vi "NavX Gyro.vi"(10 "Reset":bool, 11 "Enum":T5) -> (2 "Status":T1 {"NAVX_OP_STATUS" items=["INITIALIZING", "SELFTEST_IN_PROGRESS", "ERROR", "IMU_AUTOCAL_IN_PROGRESS", "NORMAL"]; "NAVX_CAL_STATUS" items=["IMU_CAL_STATE_MASK"=3, "IMU_CAL_INPROGRESS"=0, "IMU_CAL_ACCUMULATE"=1, "IMU_CAL_COMPLETE"=2, "MAG_CAL_COMPLETE"=4, "BARO_CAL_COMPLETE"=8]}, 3 "Angle":dbl)   [LabVIEW 2014]
uses:
  TypeDefs/SRE Enum.ctl
  navX Gyroscope/COMMON/TypeDefs/Data TypeDefs/navX Status Data.ctl
  navX Gyroscope/COMMON/TypeDefs/Value TypeDefs/navX NAVX_OP_STATUS.ctl
  navX Gyroscope/COMMON/TypeDefs/Value TypeDefs/navX NAVX_CAL_STATUS.ctl
  navX Gyroscope/COMMON/TypeDefs/Value TypeDefs/navX NAVX_SENSOR_STATUS.ctl
  navX Gyroscope/COMMON/TypeDefs/Value TypeDefs/navX Update Rate.ctl
  navX Gyroscope/COMMON/TypeDefs/Value TypeDefs/navX Interface Protocol.ctl
  <vilib>/Rock Robotics/SystemInterfaces/i2clib/i2c_bus.ctl
  navX Gyroscope/navX-MXP IMU.lvlib
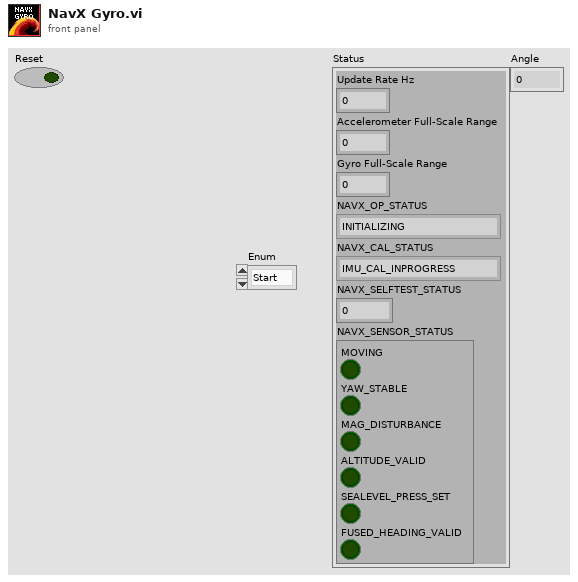
[diagram p1: front panel]
types:
  T1 = typedef "navX-MXP IMU.lvlib/navX Status Data.ctl" = cluster{"Update Rate Hz":u8, "Accelerometer Full-Scale Range":u8, "Gyro Full-Scale Range":u16, "NAVX_OP_STATUS":T2, "NAVX_CAL_STATUS":T3, "NAVX_SELFTEST_STATUS":u8, "NAVX_SENSOR_STATUS":T4}
  T2 = typedef "navX-MXP IMU.lvlib/navX NAVX_OP_STATUS.ctl" = u8
  T3 = typedef "navX-MXP IMU.lvlib/navX NAVX_CAL_STATUS.ctl" = u8
  T4 = typedef "navX-MXP IMU.lvlib/navX NAVX_SENSOR_STATUS.ctl" = cluster{"MOVING":bool, "YAW_STABLE":bool, "MAG_DISTURBANCE":bool, "ALTITUDE_VALID":bool, "SEALEVEL_PRESS_SET":bool, "FUSED_HEADING_VALID":bool}
  T5 = typedef "SRE Enum.ctl" = enum16{"Start", "Run", "End"}
  T6 = typedef "i2c_bus.ctl" = enum16{"I2C On-Board", "I2C MXP", "Invalid"}
  T7 = typedef "navX-MXP IMU.lvlib/navX Interface Protocol.ctl" = enum16{"SPI", "I2C"}
  T8 = typedef "navX-MXP IMU.lvlib/navX Update Rate.ctl" = u8
  T9 = typedef "navX-MXP IMU.lvlib/navX Device TypeDef.ctl" = cluster{"navX Interface Protocol":T7, "navX Interface Protocol TypeDefs":cluster{"SPIDevRef":T10, "I2CDevRef":T13}, "navX System Information":cluster{"Board Information":T14, "Status":T1, "Offsets":T15}, "navX Common Information":cluster{"Update Rate (4Hz-60Hz)":T8, "refnum name":string, "error":errorcluster}}
  T10 = typedef "WPI_SPIDevRef.ctl" = cluster{"DevStatus":errorcluster, "Handle":i32, "Controller":T11, "SPI Bus":T12}
  T11 = typedef "FPGA_TypedefDigitalModule.ctl" = enum16{"Controller 1"}
  T12 = typedef "spi_bus.ctl" = enum16{"SPI On-Board, CS0", "SPI On-Board, CS1", "SPI On-Board, CS2", "SPI On-Board, CS3", "SPI MXP", "Invalid"}
  T13 = typedef "WPI_I2CDevRef.ctl" = cluster{"DevStatus":errorcluster, "Controller":T11, "Device Address":u8, "Handle":i32, "I2C Bus":T6}
  T14 = typedef "navX-MXP IMU.lvlib/navX Board Information.ctl" = cluster{"WhoAmI (50 | 0x32)":u8, "Board Revision":u8, "Firmware Major Version":u8, "Firmware Minor Version":u8}
  T15 = typedef "navX-MXP IMU.lvlib/navX Offsets Data.ctl" = cluster{"Yaw":dbl, "Quat W":dbl, "Quat X":dbl, "Quat Y":dbl, "Quat Z":dbl}
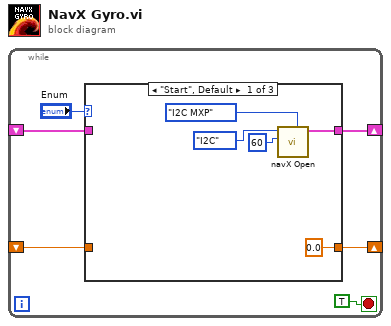
[diagram p0: block diagram]
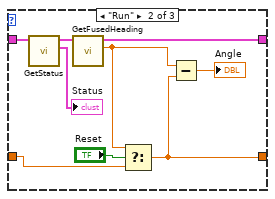
[diagram p2: hidden frame]
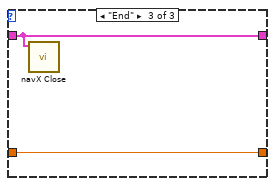
[diagram p3: hidden frame]
diagram:
  n1 = while {
    shift-right: [w4] -> _
    shift-left: _ -> [w3]
    shift-right: [w2] -> _
    shift-left: _ -> [w1]
    stop <- TRUE stop-if-true
    n2 = case shown="\"Start\", Default" "Enum" {
      tunnel: [w8 w18 w22] -> w4
      tunnel: w3 -> [_ w20 w22]
      tunnel: [0.0 ("Fused Heading") w14 w21] -> w2
      tunnel: w1 -> [_ w15 w21]
      frame "Start", Default {
        n3 = call "navX Open.vi"("I2C Bus"=i2c_bus."I2C MXP", "Update Rate (4Hz-60Hz)"=T8 60, "navX Interface Protocol"=navX_Interface_Protocol."I2C") -> ("navX Device TypeDef"=w8:T9)  [unwired: 6 in, 2 out]
      }
      frame "Run" {
        n4 = call "GetStatus.vi"("navX Device TypeDef"=w20) -> ("Status"=→"Status":T1, "navX Device TypeDef"=w19:T9)  [unwired: 8 in, 1 out]
        n5 = call "GetFusedHeading.vi"("navX Device TypeDef"=w19) -> ("Fused Heading"=w13:dbl, "navX Device TypeDef"=w18:T9)  [unwired: 8 in, 1 out]
        n6 = Select(t=w13, s="Reset", f=w15) -> (s? t:f=w14:dbl)
        n7 = Subtract(x=w13, y=w14) -> (x-y=→"Angle":dbl)
      }
      frame "End" {
        n8 = call "navX Close.vi"("navX Device TypeDef"=w22) -> ()  [unwired: 10 in, 1 out]
      }
    }
  }
